vi "Init.vi"(6 "Flags":u32=65535 format="%.0x", 8 "error in":errorcluster) -> (0 "error out":errorcluster, 3 "Return":i32)   [LabVIEW 2015, in "LibSDL2.lvlib"]
uses:
  LibSDL2.lvlib
  DLL/SDL2.dll
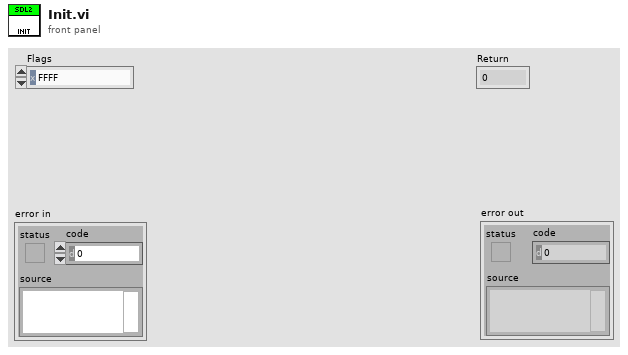
[diagram p1: front panel]
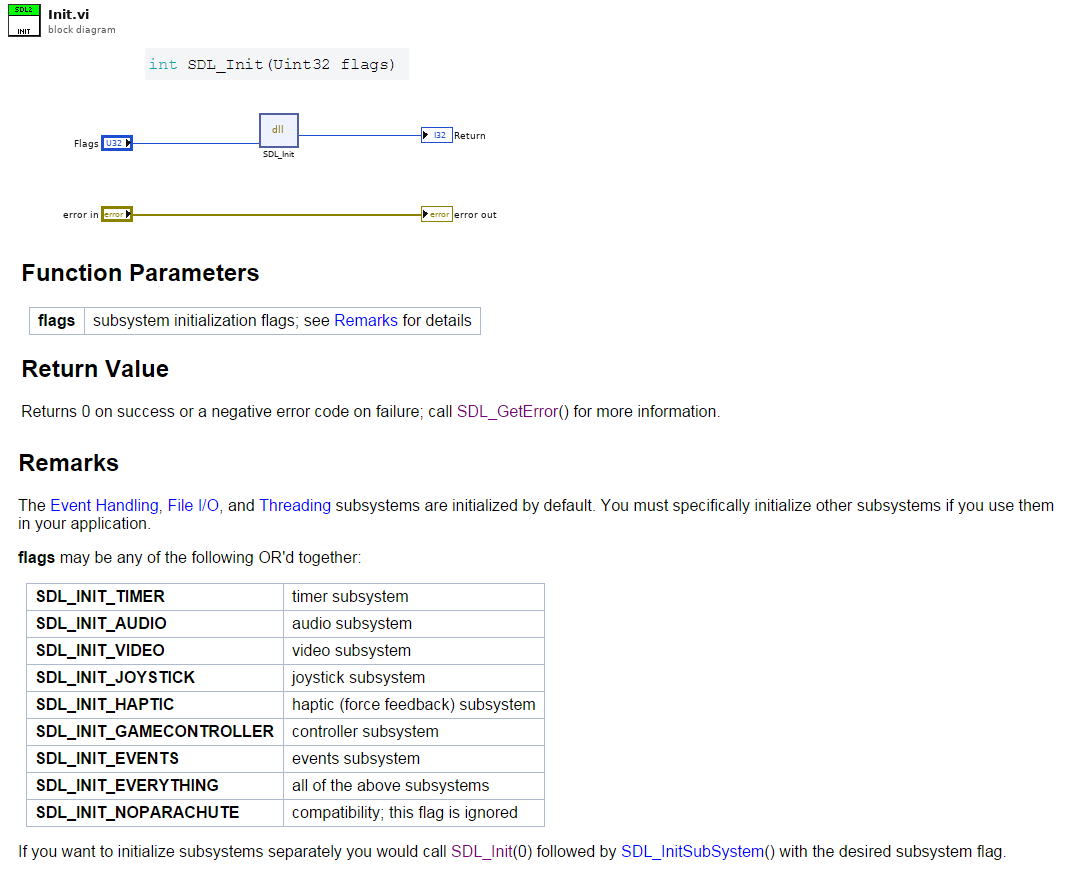
[diagram p0: block diagram]
diagram:
  n1 = dll-call lib="C:/dev/PGS/LabSDL2/Source/Libraries/LibSDL2 Wrapper/DLL/SDL2.dll" fn="SDL_Init"("flags"="Flags") -> ("return type"=→"Return":i32)  [unwired: 4 in, 2 out]
  "error out" <- "error in"
